vi "configmgr-test.vi"(8 "error in (no error)":errorcluster) -> (0 "error out":errorcluster)   [LabVIEW 2013]
uses:
  <vilib>/addons/_JKI Toolkits/Caraya/classes/Test/Test.lvclass
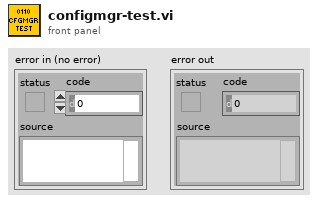
[diagram p1: front panel]
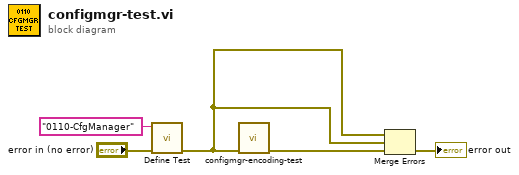
[diagram p0: block diagram]
diagram:
  n1 = call <vilib>:"Define Test.vi"("error in (no error)"="error in (no error)", "Label (VI Title)"="0110-CfgManager") -> ("error out"=w2:errorcluster)  [unwired: 9 in]
  n2 = call "configmgr-encoding-test.vi"("error in (no error)"=w2) -> ("error out"=w1:errorcluster)  [unwired: 10 in]
  n3 = Merge Errors(w2, w2, w1) -> (→"error out":errorcluster)
